vi "Remove Attribute By ID.vi"(8 "error in (no error)":errorcluster, 10 "ID":i32=-1, 11 "Attributes in":refnum<class "Attributes.lvclass">) -> (0 "error out":errorcluster, 3 "Attributes out":refnum<class "Attributes.lvclass">)   [LabVIEW 2019, in "HierDAL Library.lvlib" / "Database.lvlib" / "Repositories.lvlib" / "Attributes.lvclass"]
uses:
  Attributes.lvclass
  Attributes.lvclass/Attributes.ctl
  Database Manager Class/Database Manager.lvclass
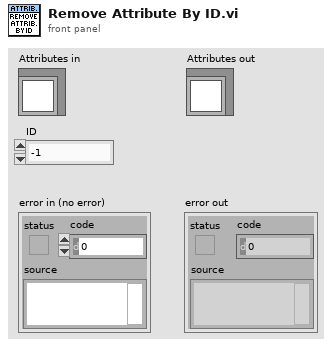
[diagram p1: front panel]
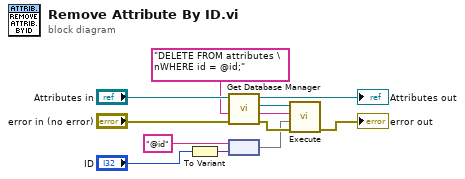
[diagram p0: block diagram]
diagram:
  n1 = To Variant(anything="ID") -> (Variant=w2:variant)
  n2 = call "Get Database Manager.vi"("error in (no error)"="error in (no error)", "Attributes in"="Attributes in") -> ("error out"=w7:errorcluster, "Database Manager"=w6:refnum<class "Database Manager.lvclass">, "Attributes out"=→"Attributes out":refnum<class "Attributes.lvclass">)  [unwired: 7 in]
  n3 = node("@id" ("key"), w2) -> (w1:map{string, variant})
  n4 = call-dynamic "Execute.vi"("error in (no error)"=w7, "Parameters"=w1, "Query"="DELETE FROM attributes \nWHERE id = @id;", "Database Manager in"=w6) -> ("error out"=→"error out":errorcluster)  [unwired: 5 in, 2 out]
